vi "CloseEthConnection.vi"(8 "error in (no error)":errorcluster, 11 "connection ID":refnum<k5>) -> (0 "error out":errorcluster)   [LabVIEW 2015, in "VIPM2.lvlib"]
uses:
  VIPM2.lvlib
panel:
  out "bytes written":i32
  # "Close Ethernet connection"
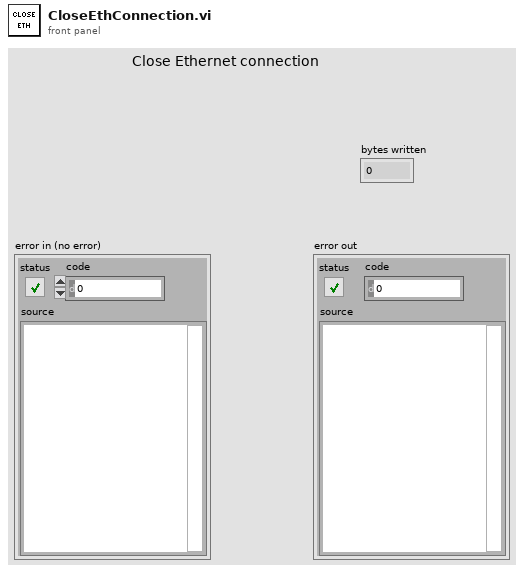
[diagram p1: front panel]
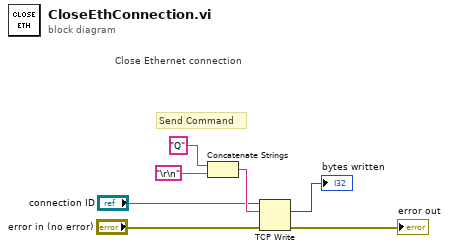
[diagram p0: block diagram]
diagram:
  # "Send Command"
  # "Close Ethernet connection"
  n1 = Concatenate Strings("Q" ("string"), "\r\n") -> (w6:string)
  n2 = TCP Write(connection ID="connection ID", data in=w6, error in (no error)="error in (no error)") -> (bytes written=→"bytes written":i32, error out=→"error out":errorcluster)  [unwired: 1 in, 1 out]
